vi "Öffnen.vi"(8 "Error In":errorcluster caption="Fehler (Eingang)") -> (0 "Error Out":errorcluster caption="Fehler (Ausgang)", 3 "Verbindungs-ID":refnum<k16>)   [LabVIEW 2019, in "Thermostat Treiber.lvlib"]
uses:
  Thermostat Treiber.lvlib
  SubVIs/Simulation Share.vi
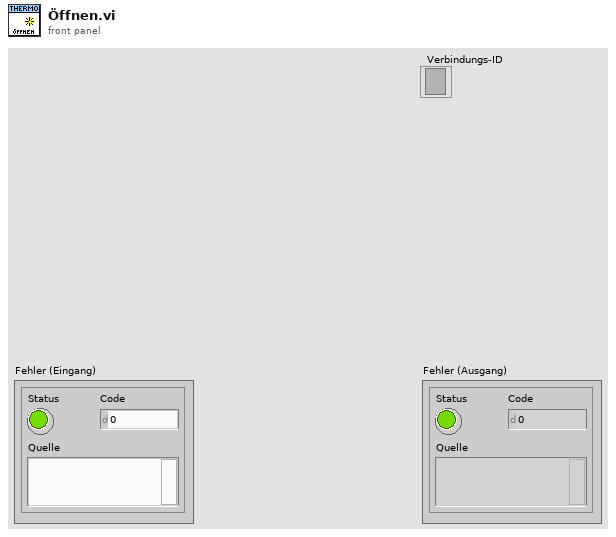
[diagram p1: front panel]
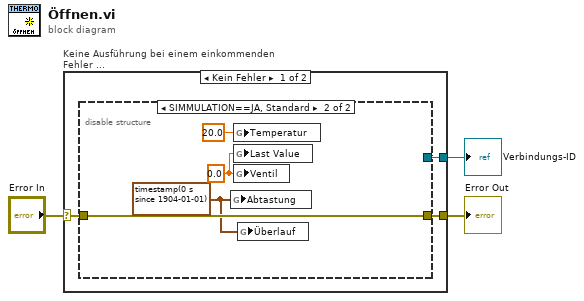
[diagram p0: block diagram]
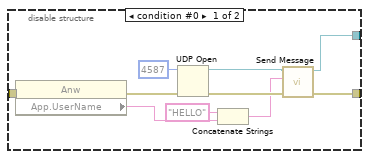
[diagram p2: hidden frame]
diagram:
  n1 = case "Keine Ausführung bei einem einkommenden Fehler ..." shown="Kein Fehler" "Error In" {
    selector: "Error In" -> [w4 w21]
    tunnel: [w5 w21] -> w2
    tunnel: [w6 _] -> w1
    frame No Error {
      n2 = disable-structure shown="SIMMULATION==JA, Standard" {
        disable-tunnel: [w16 _] -> w6
        disable-tunnel: [w15 w20] -> w5
        disable-tunnel: w4 -> [w14 w20]
        frame condition #0 {
          n3 = property class="Anw"(error in=w14) -> (error out=w9:errorcluster, "App.UserName"=w7:string)  [unwired: 1 in, 1 out]
          n4 = UDP Open(8:w9, 11:u16 4587 ("Port")) -> (port=w11:refnum<k16>, 0:w12:errorcluster)  [unwired: 3 in, 1 out]
          n5 = Concatenate Strings("HELLO" ("Nachricht"), w7) -> (w8:string)
          n6 = call "Send Message.vi"("Error In"=w12, "Nachricht"=w8, "Verbindungs-ID in"=w11) -> ("Error Out"=w15:errorcluster, "Verbindungs-ID out"=w16:refnum<k16>)  [unwired: 7 in]
        }
        frame condition #1 (active) {
          w17 = timestamp(0 s since 1904-01-01) ("Abtastung")
          w19 = 0.0 ("Ventil")
          n7 = global write "Simulation Share.vi" "Abtastung"(w17) -> ()
          n8 = global write "Simulation Share.vi" "Temperatur"(20.0 ("Temperatur")) -> ()
          n9 = global write "Simulation Share.vi" "Last Value"(w19) -> ()
          n10 = global write "Simulation Share.vi" "Ventil"(w19) -> ()
          n11 = global write "Simulation Share.vi" "Überlauf"(w17) -> ()
        }
      }
    }
    frame Error {
    }
  }
  "Error Out" <- w2
  "Verbindungs-ID" <- w1
